vi "Read Local Msg Set.vi"(11 "Core Actor in":refnum<class "Core Actor.lvclass">) -> (2 "Local Msg Set":T1)   [LabVIEW 2025, in "jettl.lvlib" / "Core Actor.lvlib" / "Core Actor.lvclass"]
uses:
  Core Actor.lvclass
  Msg Set.ctl
  Msg/Msg.lvclass
  Core Actor.lvclass/Core Actor.ctl
  jettl.lvlib
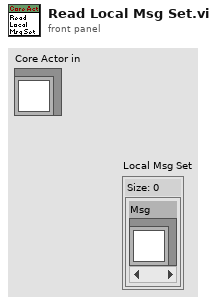
[diagram p1: front panel]
types:
  T1 = typedef "jettl.lvlib/Msg Set.ctl" = set{refnum<class "Msg.lvclass">}
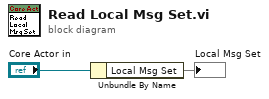
[diagram p0: block diagram]
diagram:
  n1 = Unbundle By Name("Core Actor in") -> ("Local Msg Set"=→"Local Msg Set":T1)
